vi "Set Local Chassis Name.vi"(8 "error in":errorcluster, 10 "name":string, 11 "chassis ref in":T1 format="%.0x") -> (0 "error out":errorcluster, 3 "chassis ref out":T1 format="%.0x")   [LabVIEW 2020, in "Scan Engine Scripting.lvlib"]
doc: "Writes <B>name</B> into the provided chassis reference as the the local chassis name."
uses:
  Scan Engine Scripting.lvlib
  <vilib>/NI VeriStand/Custom Device API/Custom Device Item Ref.ctl
  <vilib>/NI VeriStand/Custom Device API/Custom Device API.lvlib
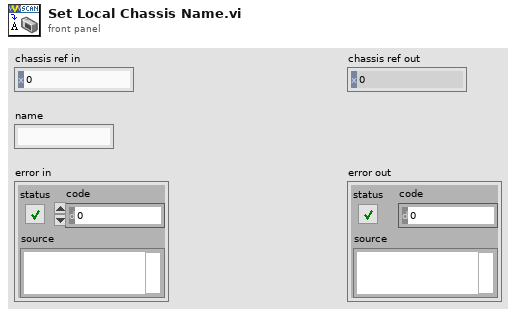
[diagram p1: front panel]
types:
  T1 = typedef "Custom Device API.lvlib/Custom Device Item Ref.ctl" = u64
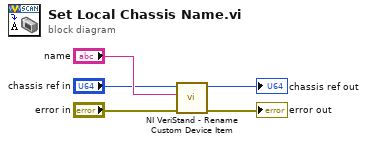
[diagram p0: block diagram]
diagram:
  n1 = call <vilib>:"NI VeriStand - Rename Custom Device Item.vi"("error in (no error)"="error in", "New Name"="name", "Item Ref in"="chassis ref in") -> ("error out"=→"error out":errorcluster, "Item Ref out"=→"chassis ref out":T1)  [unwired: 1 in, 6 out]
